vi "main.vi"() -> ()   [LabVIEW 2019]
uses:
  Controls/semafor.ctl
  Controls/Estats.ctl
panel:
  in  "reset":bool
  out "Semafor":T1
  out "pedestrian":bool
  in  "Boolean":bool
  in  "stop":bool
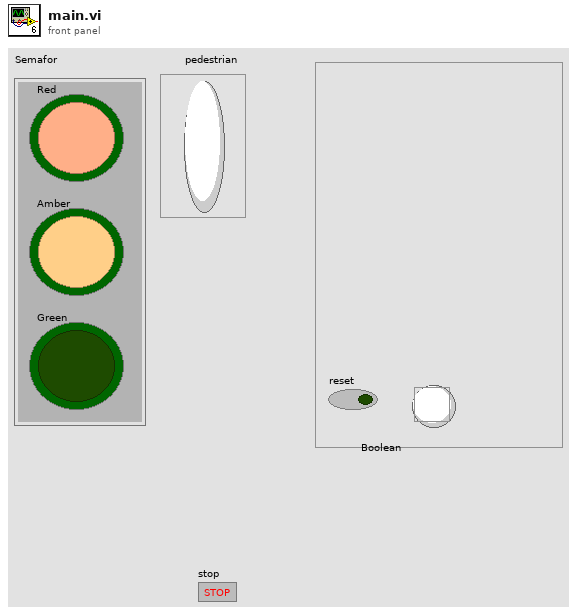
[diagram p1: front panel]
types:
  T1 = typedef "semafor.ctl" = cluster{"Red":bool, "Amber":bool, "Green":bool}
  T2 = typedef "Estats.ctl" = enum16{"Init", "Green", "Amber-red", "red", "amber"}
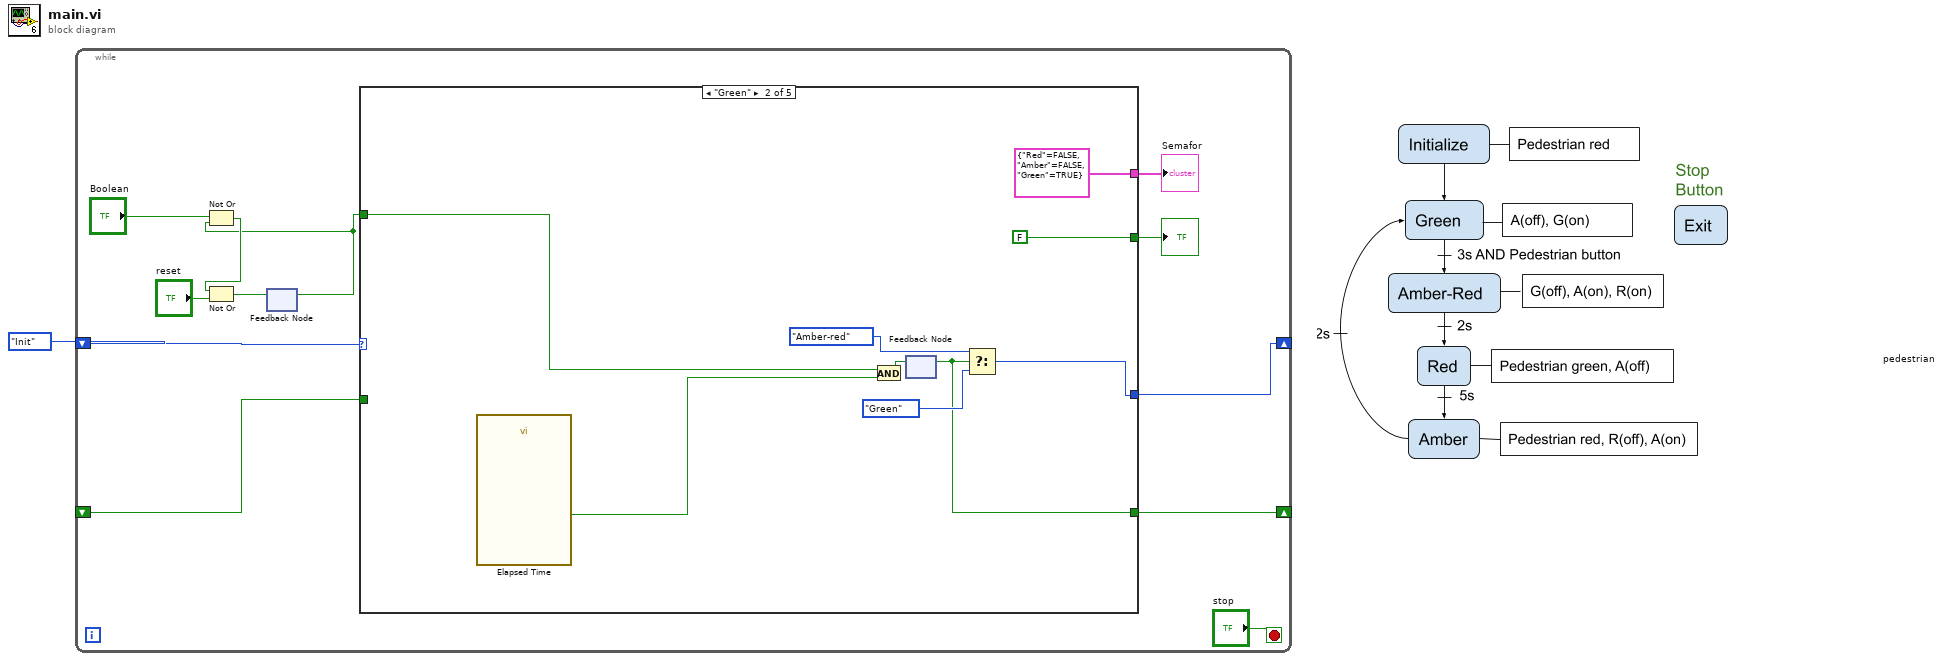
[diagram p0: block diagram]
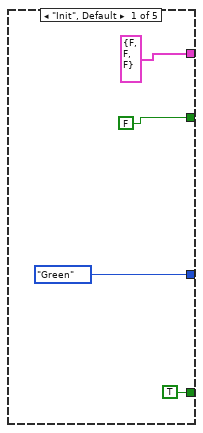
[diagram p2: hidden frame]
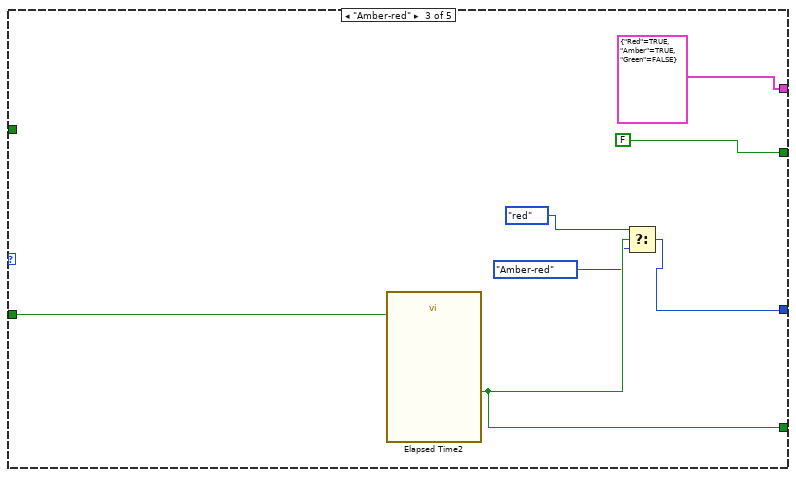
[diagram p3: hidden frame]
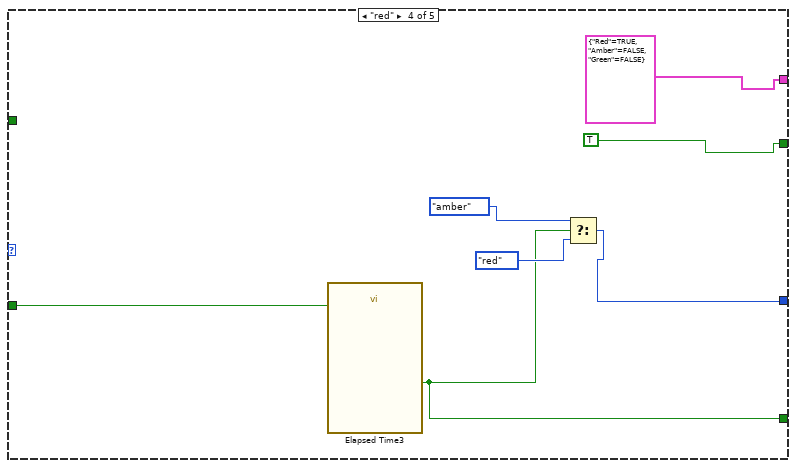
[diagram p4: hidden frame]
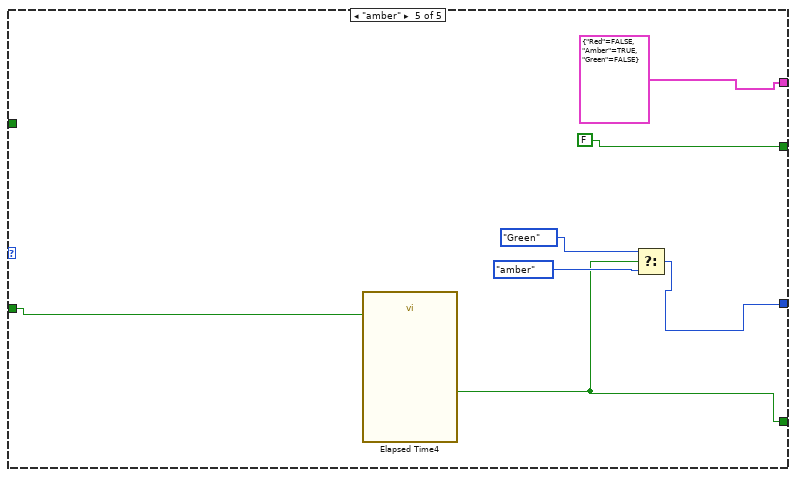
[diagram p5: hidden frame]
diagram:
  n1 = while {
    shift-right: [w12] -> _
    shift-left: _ -> [w11]
    shift-right: [w7] -> _
    shift-left: Estats."Init" ("Enum") -> [w8]
    stop <- "stop" stop-if-true
    n2 = feedback #1() -> (w3:bool)  [unwired: 1 in]
    n3 = Not Or(1:w3, 2:"Boolean") -> (0:w6:bool)
    n4 = Not Or(1:"reset", 2:w6) -> (0:w4:bool)
    n5 = feedback-in #1(w4) -> ()
    n6 = case shown="\"Green\"" w8 {
      tunnel: [Estats."Green" ("Enum") w23 w33 w38 w45] -> w7
      tunnel: [TRUE ("Time has Elapsed") w19 w31 w37 w44] -> w12
      tunnel: w11 -> [_ _ w29 w36 w43]
      tunnel: [T1 {"Red"=FALSE, "Amber"=FALSE, "Green"=FALSE} ("Semafor") T1 {"Red"=FALSE, "Amber"=FALSE, "Green"=TRUE} ("Semafor") T1 {"Red"=TRUE, "Amber"=TRUE, "Green"=FALSE} ("Semafor") T1 {"Red"=TRUE, "Amber"=FALSE, "Green"=FALSE} ("Semafor") T1 {"Red"=FALSE, "Amber"=TRUE, "Green"=FALSE} ("Semafor")] -> w10
      tunnel: [FALSE ("pedestrian") FALSE ("pedestrian") FALSE ("pedestrian") TRUE ("pedestrian") FALSE ("pedestrian")] -> w9
      tunnel: w3 -> [_ w18 _ _ _]
      frame "Init", Default {
      }
      frame "Green" {
        n7 = call "Elapsed Time"() -> ("Time has Elapsed"=w24:bool)  [unwired: 12 in, 7 out]
        n8 = And(x=w18, y=w24) -> (x .and. y?=w20:bool)
        n9 = feedback-in #2(w20) -> ()
        n10 = feedback #2() -> (w19:bool)  [unwired: 1 in]
        n11 = Select(t=Estats."Amber-red" ("Enum"), s=w19, f=Estats."Green" ("Enum")) -> (s? t:f=w23:T2)
      }
      frame "Amber-red" {
        n12 = call "Elapsed Time2"("Reset"=w29) -> ("Time has Elapsed"=w31:bool)  [unwired: 11 in, 7 out]
        n13 = Select(t=Estats."red" ("Enum"), s=w31, f=Estats."Amber-red" ("Enum")) -> (s? t:f=w33:T2)
      }
      frame "red" {
        n14 = call "Elapsed Time3"("Reset"=w36) -> ("Time has Elapsed"=w37:bool)  [unwired: 11 in, 7 out]
        n15 = Select(t=Estats."amber" ("Enum"), s=w37, f=Estats."red" ("Enum")) -> (s? t:f=w38:T2)
      }
      frame "amber" {
        n16 = call "Elapsed Time4"("Reset"=w43) -> ("Time has Elapsed"=w44:bool)  [unwired: 11 in, 7 out]
        n17 = Select(t=Estats."Green" ("Enum"), s=w44, f=Estats."amber" ("Enum")) -> (s? t:f=w45:T2)
      }
    }
    "Semafor" <- w10
    "pedestrian" <- w9
  }
